vi "PulseGeneration.vi"() -> (1 "waveform":dbl[](array[numeric]), 3 "tRange":dbl)   [LabVIEW 2015]
uses:
  <vilib>/imath/engines/lvmath2/RunTimeEngine/BuiltInFunctions/nextpowerof2/NIMS_nextpowerof2(GS).vi
  <instcachedir>/0/NIMS_nextpowerof2(GS)_B42BF357393E46BBAF4FDD53A40AE50C.lvgen/NIMS_nextpowerof2(GS)_B42BF357393E46BBAF4FDD53A40AE50C_000.vi
  <vilib>/imath/engines/lvmath2/RunTimeEngine/RangeToken/NIMS_Range.vi
  <instcachedir>/0/NIMS_Range_D919CC09935940E88F755EC1C6F49AC1.lvgen/NIMS_Range_D919CC09935940E88F755EC1C6F49AC1_000.vi
  <vilib>/imathl/engines/lvmath/Functions/Error Handling/Create Error.vi
  <vilib>/imath/engines/lvmath2/RunTimeEngine/ArithmeticOperatorToken/NIMS_ArithmeticOperator_times.vi
  <instcachedir>/0/NIMS_ArithmeticOperator_times_DF26C4080E2A467BA28C929B8CF31953.lvgen/NIMS_ArithmeticOperator_times_DF26C4080E2A467BA28C929B8CF31953_003.vi
  <vilib>/imath/engines/lvmath2/RunTimeEngine/BuiltInFunctions/abs/NIMS_abs(signed).vi
  <instcachedir>/0/NIMS_abs(signed)_C4FCB8E6058B49B797C7C8D53CA5F6EC.lvgen/NIMS_abs(signed)_C4FCB8E6058B49B797C7C8D53CA5F6EC_006.vi
  <vilib>/imath/engines/lvmath2/RunTimeEngine/BuiltInFunctions/max/1 input/NIMS_max(RV).vi
  <instcachedir>/0/NIMS_max(RV)_237633DB1D604D5BA7001287DF3C7957.lvgen/NIMS_max(RV)_237633DB1D604D5BA7001287DF3C7957_000.vi
  <vilib>/imath/engines/lvmath2/RunTimeEngine/NodeEndStatement/NIMS_NodeEndStatement_Output.vi
  <instcachedir>/0/NIMS_NodeEndStatement_Output_53EC0D466D134D7ABD903AC30B43404B.lvgen/NIMS_NodeEndStatement_Output_53EC0D466D134D7ABD903AC30B43404B_001.vi
  <instcachedir>/0/NIMS_NodeEndStatement_Output_53EC0D466D134D7ABD903AC30B43404B.lvgen/NIMS_NodeEndStatement_Output_53EC0D466D134D7ABD903AC30B43404B_005.vi
  <vilib>/imath/engines/lvmath2/RunTimeEngine/ErrorHandling/NIMS_Finalize Error.vi
panel:
  in  "FWHM (us)":dbl=1.0
  in  "Number of data points":u32=131072 min=2 max=131072 step=1
  in  "f0 (Hz)":dbl=80.0
  out "XY Graph 2":cluster{dbl[], "Windowed X":dbl[]}(graph)
  out "Effective N value (nexpow2)":u32=131072
  in  "OK Button":bool
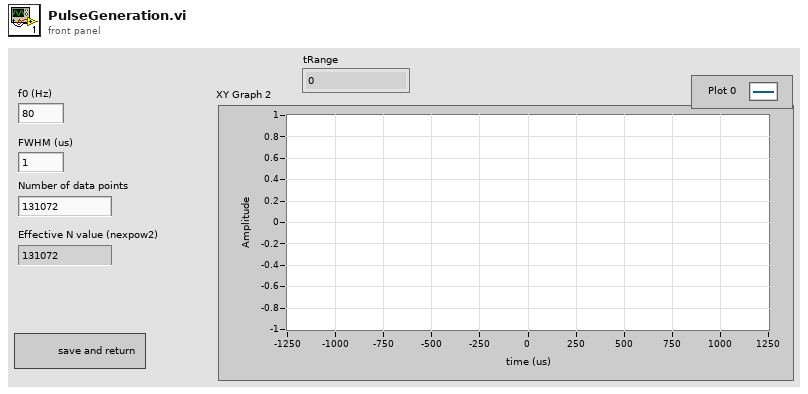
[diagram p1: front panel]
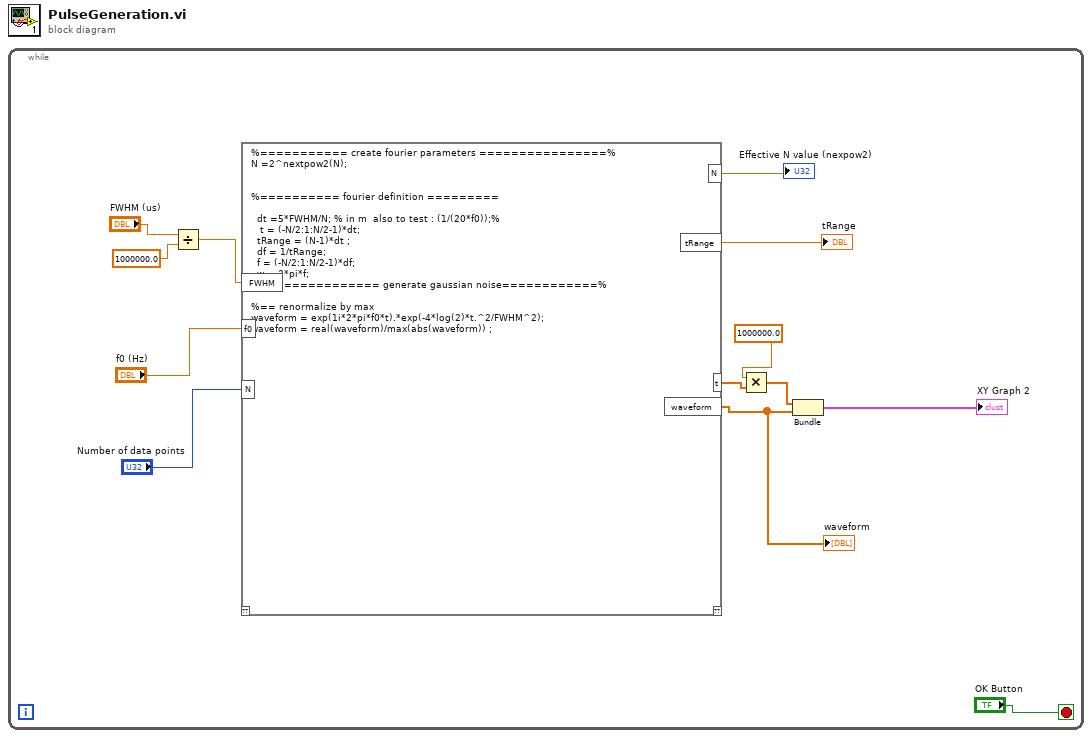
[diagram p0: block diagram]
diagram:
  n1 = while {
    stop <- "OK Button" stop-if-true
    n2 = Divide(x="FWHM (us)", y=1000000.0) -> (x/y=w5:dbl)
    n3 = mathscript code="%=========== create fourier parameters ================%\nN =2^nextpow2(N);\n\n\n%========== fourier definition =========\n\n  dt =5*FWHM/N; % in m  also to test : (1/(20*f0));%\n   t = (-N/2:1:N/2-1)*dt;\n  tRange = (N-1)*dt ;\n  df = 1/tRange;\n  f = (-N/2:1:N/2-1)*df;\n  w = 2*pi*f;\n%=============== generate gaussian noise============%\n\n%== renormalize by max\nwaveform = exp(1i*2*pi*f0*t).*exp(-4*log(2)*t.^2/FWHM^2);\nwaveform = real(waveform)/max(abs(waveform)) ;"("f0"="f0 (Hz)", "FWHM"=w5, "N"="Number of data points") -> ("t"=w4:dbl[], "waveform"=w11:dbl[], "N"=→"Effective N value (nexpow2)":dbl, "tRange"=→"tRange":dbl)  [unwired: 1 in, 1 out]
    "waveform" <- w11
    n4 = Multiply(x=1000000.0, y=w4) -> (x*y=w2:dbl[])
    n5 = Bundle(w2, "waveform"=w11) -> (→"XY Graph 2":cluster{dbl[], "waveform":dbl[]})  [unwired: 1 in]
  }
